vi "visa_loop_counter.vi"(8 "Error In":errorcluster, 11 "Finished Late? [i-1]":bool) -> (0 "Error Out":errorcluster, 1 "Last millisecond time in":u32, 2 "On time counter buffer in":i32, 3 "Late counter buffer in":i32, 5 "Loop cycle rate":u32)   [LabVIEW 2019]
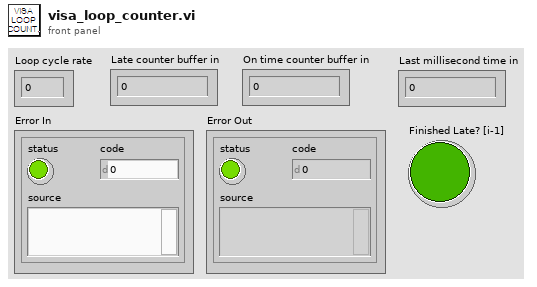
[diagram p1: front panel]
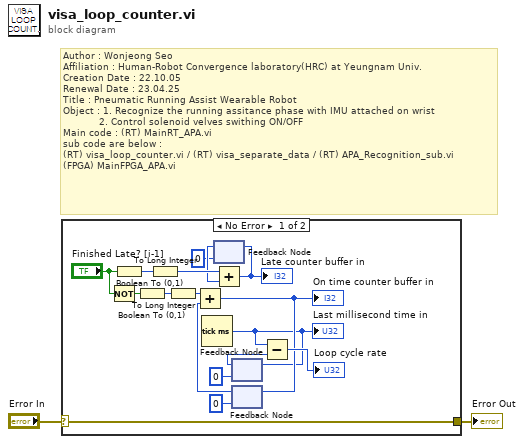
[diagram p0: block diagram]
diagram:
  # "Author : Wonjeong Seo\nAffiliation : Human-Robot Convergence laboratory(HRC) at Yeungnam Univ.\nCreation Date : 22.10.05\nRenewal Date : 23.04.25\nTitle : Pneumatic Running Assist Wearable Robot\nObject : 1. Recognize the running assitance phase with IMU attached on wrist\n            2. Control solenoid velves swithing ON/OFF\nMain code : (RT) MainRT_APA.vi\nsub code are below :\n(RT) visa_loop_counter.vi / (RT) visa_separate_data / (RT) APA_Recognition_sub.vi\n(FPGA) MainFPGA_APA.vi"
  n1 = case shown="No Error" "Error In" {
    selector: "Error In" -> [w16 w20]
    tunnel: [w16 w20] -> w1
    frame No Error {
      n2 = Not(x="Finished Late? [i-1]") -> (.not. x?=w12:bool)
      n3 = Boolean To (0,1)(Boolean="Finished Late? [i-1]") -> (0, 1=w18:i16)
      n4 = Boolean To (0,1)(Boolean=w12) -> (0, 1=w11:i16)
      n5 = To Long Integer(number=w18) -> (32bit integer=w17:i32)
      n6 = To Long Integer(number=w11) -> (32bit integer=w10:i32)
      n7 = Tick Count (ms)() -> (millisecond timer value=w3:u32)
      "Last millisecond time in" <- w3
      n8 = feedback #1(0) -> (w14:i32)
      n9 = Add(x=w17, y=w14) -> (x+y=w15:i32)
      "Late counter buffer in" <- w15
      n10 = feedback-in #1(w15) -> ()
      n11 = feedback #2(u32 0) -> (w8:u32)
      n12 = feedback-in #2(w3) -> ()
      n13 = feedback #3(0) -> (w6:i32)
      n14 = Add(x=w10, y=w6) -> (x+y=w7:i32)
      "On time counter buffer in" <- w7
      n15 = feedback-in #3(w7) -> ()
      n16 = Subtract(x=w3, y=w8) -> (x-y=→"Loop cycle rate":u32)
    }
    frame Error {
    }
  }
  "Error Out" <- w1
